vi "AuMT8852B Block Write.vi"(5 "Data (\"\")":string, 7 "Command (\"\")":string, 8 "error in (no error)":errorcluster, 11 "VISA Session":refnum<visa-resource-name>) -> (0 "error out":errorcluster, 3 "VISA Session out":refnum<visa-resource-name>)   [LabVIEW 2017]
doc: "Anritsu MT8852B Bluetooth Tester\n\nWrites binary data to the instrument in Arbitrary Block format:\n#<width of byte count><byte count><data>.\n\nINPUTS\nCommand - Command to precede block data\nData - contents of the block data."
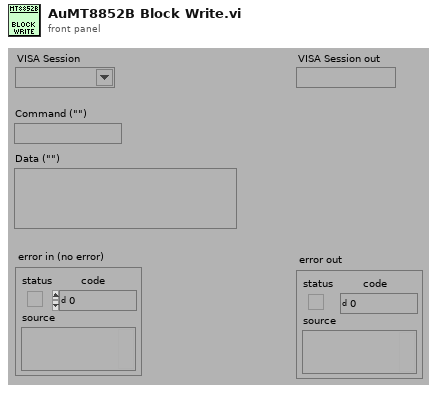
[diagram p1: front panel]
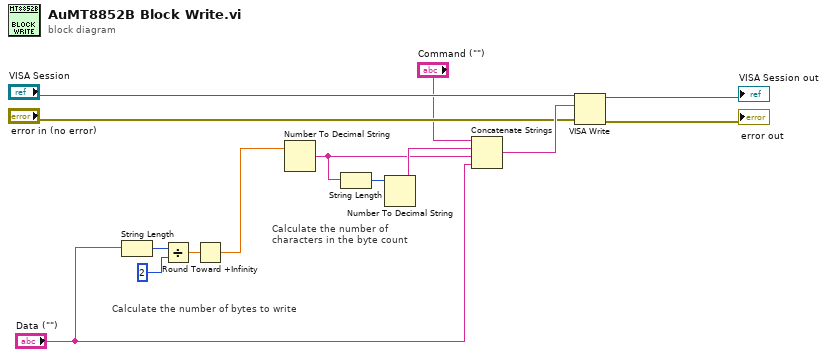
[diagram p0: block diagram]
diagram:
  # "Calculate the number of \ncharacters in the byte count"
  # "Calculate the number of bytes to write"
  n1 = String Length(string="Data (\"\")") -> (length=w14:i32)
  n2 = Divide(x=w14, y=2) -> (x/y=w12:dbl)
  n3 = Round Toward +Infinity(x=w12) -> (ceil(x): smallest int >= x=w11:dbl)
  n4 = Number To Decimal String(number=w11) -> (decimal integer string=w8:string)  [unwired: 1 in]
  n5 = String Length(string=w8) -> (length=w10:i32)
  n6 = Number To Decimal String(number=w10) -> (decimal integer string=w9:string)  [unwired: 1 in]
  n7 = Concatenate Strings("Command (\"\")", w9, w8, "Data (\"\")") -> (w7:string)
  n8 = VISA Write(VISA resource name="VISA Session", write buffer=w7, error in (no error)="error in (no error)") -> (VISA resource name out=→"VISA Session out":refnum<visa-resource-name>, error out=→"error out":errorcluster)  [unwired: 1 out]
